vi "convert voltages.vi"(8 "error in (no error)":errorcluster, 10 "1x160 Voltage Map":dbl[](array[numeric]), 11 "BMC in":refnum<class "BMC.lvclass">) -> (0 "error out":errorcluster, 2 "Voltage array out":u16[](array[numeric]), 3 "BMC out":refnum<class "BMC.lvclass">)   [LabVIEW 2012, in "BMC.lvclass"]
uses:
  BMC.lvclass
  BMC.lvclass/BMC.ctl
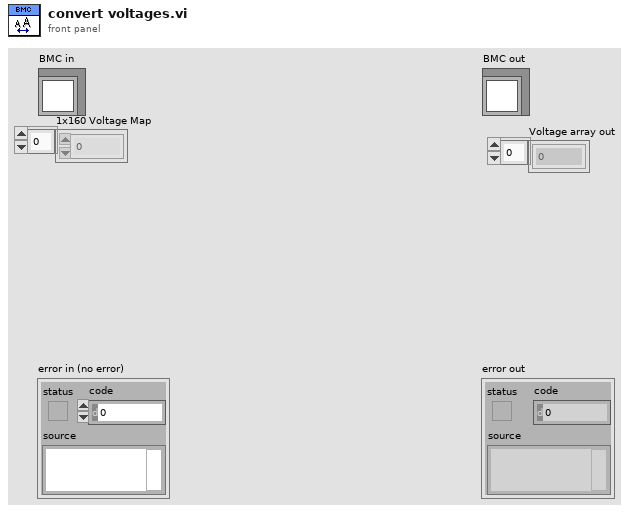
[diagram p1: front panel]
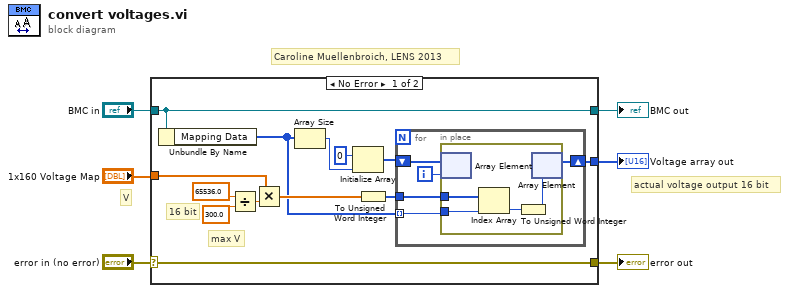
[diagram p0: block diagram]
diagram:
  # "actual voltage output 16 bit"
  # "V"
  # "Caroline Muellenbroich, LENS 2013"
  n1 = case shown="No Error" "error in (no error)" {
    selector: "error in (no error)" -> [w19 w30]
    tunnel: [w19 w30] -> w5
    tunnel: [w18 w29] -> w3
    tunnel: "BMC in" -> [w18 w29]
    tunnel: [w11 _] -> w2
    tunnel: "1x160 Voltage Map" -> [w8 _]
    frame No Error {
      # "16 bit"
      # "max V"
      n2 = Unbundle By Name(w18) -> ("Mapping Data"=w7:i32[])
      n3 = Divide(x=65536.0 ("y"), y=300.0 ("x")) -> (x/y=w17:dbl)
      n4 = Multiply(x=w8, y=w17) -> (x*y=w10:dbl[])
      n5 = Array Size(array=w7) -> (size(s)=w13:i32)
      n6 = Initialize Array(u16 0 ("element"), w13) -> (w12:u16[])
      n7 = To Unsigned Word Integer(number=w10) -> (unsigned 16bit integer=w9:u16[])
      n8 = for {
        shift-right: [w20] -> w11
        shift-left: w12 -> [w21]
        tunnel: w9 -> [w23]
        tunnel: w7 -> [w22] mode=indexing
        i -> [w24]
        n9 = in-place {
          in-place-border: w23 -> [w26]
          in-place-border: w22 -> [w28]
          n10 = in-place-array #1(w21, w24) -> ()  [unwired: 1 out]
          n11 = Index Array(array=w26, index=w28) -> (element=w25:u16)
          n12 = To Unsigned Word Integer(number=w25) -> (unsigned 16bit integer=w27:u16)
          n13 = in-place-array #1(w27) -> (w20:u16[])  [unwired: 1 out]
        }
      }
    }
    frame Error {
    }
  }
  "error out" <- w5
  "BMC out" <- w3
  "Voltage array out" <- w2
